vi "NI VeriStand - Load Runtime Configuration File.vi"(8 "Error in":errorcluster, 11 "Runtime Configuration File":string) -> (0 "Error out":errorcluster, 2 "Base Section ID":u64, 3 "Runtime Configuration Ref":refnum<k39>)   [LabVIEW 2025, in "Runtime Configuration File API.lvlib"]
uses:
  Runtime Configuration File API.lvlib
  C:/NetCoreDLL/NationalInstruments.VeriStand.SystemDefinitionAPI.dll
  NetCoreDLL/NationalInstruments.VeriStand.SystemDefinitionAPI.dll
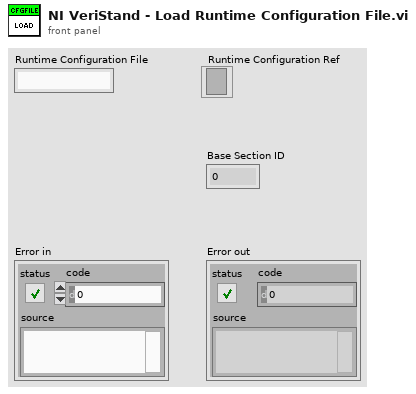
[diagram p1: front panel]
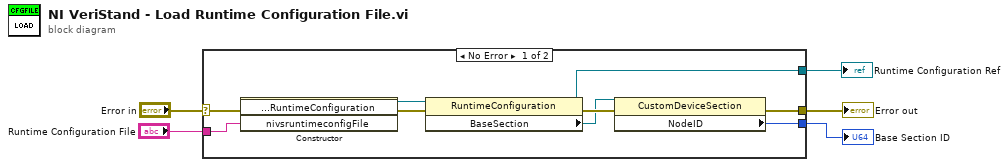
[diagram p0: block diagram]
diagram:
  n1 = case shown="No Error" "Error in" {
    selector: "Error in" -> [w14 w15]
    tunnel: [w11 w15] -> w4
    tunnel: "Runtime Configuration File" -> [w10 _]
    tunnel: [w7 _] -> w2
    tunnel: [w6 _] -> w1
    frame No Error {
      n2 = constructor class="RuntimeConfiguration"(error in=w14, "nivsruntimeconfigFile"=w10) -> (reference out=w8:refnum<k39>, error out=w12:errorcluster)  [unwired: 2 in, 2 out]
      n3 = property class="RuntimeConfiguration"(reference=w8, error in=w12) -> (reference out=w7:refnum<k39>, error out=w13:errorcluster, "BaseSection"=w9:refnum<k39>)
      n4 = property class="CustomDeviceSection"(reference=w9, error in=w13) -> (error out=w11:errorcluster, "NodeID"=w6:u64)  [unwired: 1 out]
    }
    frame Error {
    }
  }
  "Error out" <- w4
  "Runtime Configuration Ref" <- w2
  "Base Section ID" <- w1
